vi "get hydrolysis fractions.vi"(8 "error in (no error)":errorcluster) -> (0 "error out":errorcluster, 3 "function return":string)   [LabVIEW 2019, in "libSimulationControl.lvlib"]
doc: "const char* get_hydrolysis_fractions();"
uses:
  libSimulationControl.lvlib
  libSimulationControl.so
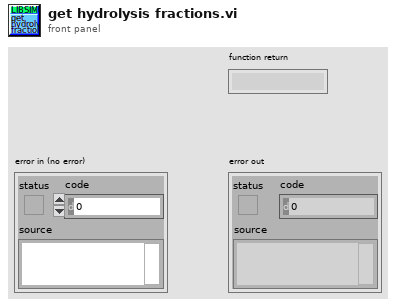
[diagram p1: front panel]
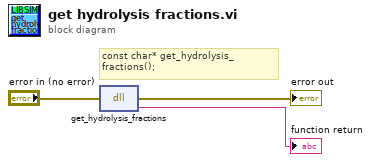
[diagram p0: block diagram]
diagram:
  # "const char* get_hydrolysis_fractions();"
  n1 = dll-call lib="home/paul/Schreibtisch/Biogas_plant_setup/LabView/lib/libSimulationControl/libSimulationControl.*" fn="get_hydrolysis_fractions"(error in="error in (no error)") -> (error out=→"error out":errorcluster, →"function return":string)  [unwired: 2 in, 1 out]
